vi "Initialization_UI.vi"(8 "error in (no error)":errorcluster, 11 "ZenGage v3.0 UI in":refnum<class "ZenGage v3.0 UI.lvclass">) -> (0 "error out":errorcluster, 3 "ZenGage v3.0 UI out":refnum<class "ZenGage v3.0 UI.lvclass">)   [LabVIEW 2015, in "ZenGage v3.0 UI.lvclass"]
uses:
  ZenGage v3.0 UI.lvclass
  ZenGage v3.0 UI.lvclass/ZenGage v3.0 UI.ctl
  <vilib>/Utility/miscctls.llb/LVRowAndColumnTypeDef.ctl
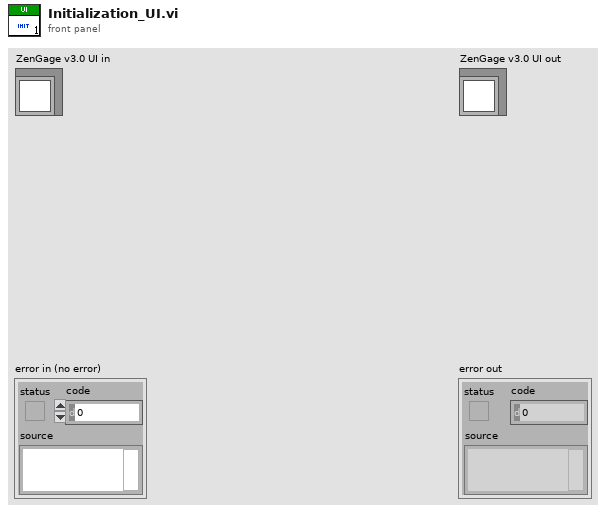
[diagram p1: front panel]
types:
  T1 = enum8{"Enabled", "Disabled", "Disabled and Grayed Out"}
  T2 = enum32{"Edit Tolerance Limits1", "Inspection", "Diagnostics", "Other Diagnostics"}
  T3 = enum32{"Analytics", "Blank", "Diagnostics", "Run", "Edit Tolerance Settings"}
  T4 = typedef "LVRowAndColumnTypeDef.ctl" = cluster{"Row":i32, "Column":i32}
  T5 = typedef "ZenGage v3.0 UI.lvclass/UI JSON read cluster.ctl" = cluster{"UIParameters":cluster{"SpecificationVersion":string, "Title":string, "NumberOfImagesToBeDisplayed":dbl, "ImageCountWindow":dbl, "FontName":string, "FontSize":dbl, "CustomerLogoFilePath":string, "ZentronLogoFilePath":string, "CompatibleSoftwareVersions":string[], "CameraLabelMapping":cluster{"CameraName":string, "ImageLabel":string}[], "ImageIndicatorLayouts":cluster{"NumberOfImageIndicators":dbl, "ImageSpecificData":cluster{"Width":dbl, "Left":dbl, "Top":dbl, "ImagePercentage":cluster{"Height":dbl, "Widthcorrection":i64, "Heightcorrection":i64, "Leftcorrection":dbl, "Topcorrection":dbl}, "StringPercentage":cluster{"Height":dbl, "Widthcorrection":i64, "Heightcorrection":dbl, "Leftcorrection":dbl, "Topcorrection":dbl}}[]}[], "SoftwareButtonLabels":cluster{"SelectLabel":string, "RunLabel":string, "PauseLabel":string, "StopLabel":string}, "DiagnosticsParameters":cluster{"CameraOpticsDiagnostics":cluster{"Label":string, "CameraLabelsList":cluster{"CameraName":string, "ImageLabel":string}[]}, "ArduinoDiagnostics":cluster{"Label":string}, "GuideMotor":cluster{"Label":string}, "ReelerMotor":cluster{"Label":string}, "TowerLamp":cluster{"Label":string}, "TriggerSensor":cluster{"Label":string, "SensorsList":cluster{"SensorName":string, "LabelName":string}[]}, "HardwareButtonDiagnostics":cluster{"Label":string}}, "DieIdParameters":cluster{"DefaultDieId":string, "DieIdsList":string[]}, "EventReasonsList":cluster{"Pause":string[], "Stop":string[], "FailPause":string[], "DefaultEventReason":string}, "StampingMachineIds":string[], "ErrorPopupStrings":cluster{"ErrorCode":string, "ErrorString":string}[]}}
  T6 = cluster{"CameraOpticsDiagnostics":cluster{"Label":string, "CameraLabelsList":cluster{"CameraName":string, "ImageLabel":string}[]}, "ArduinoDiagnostics":cluster{"Label":string}, "GuideMotor":cluster{"Label":string}, "ReelerMotor":cluster{"Label":string}, "TowerLamp":cluster{"Label":string}, "TriggerSensor":cluster{"Label":string, "SensorsList":cluster{"SensorName":string, "LabelName":string}[]}, "HardwareButtonDiagnostics":cluster{"Label":string}}
  T7 = cluster{"Diagnostics names":cluster{"Main diagnostics":string[], "Sub diagnostics names":cluster{"Camera optics":string[], "Trigger sensor":string[]}}, "Diagnostics labels":cluster{"Main diagnostics":string[], "Sub diagnostics names":cluster{"Camera optics":string[], "Trigger sensor":string[]}}}
  T8 = typedef "IMAQ Image.ctl" = refnum<image>
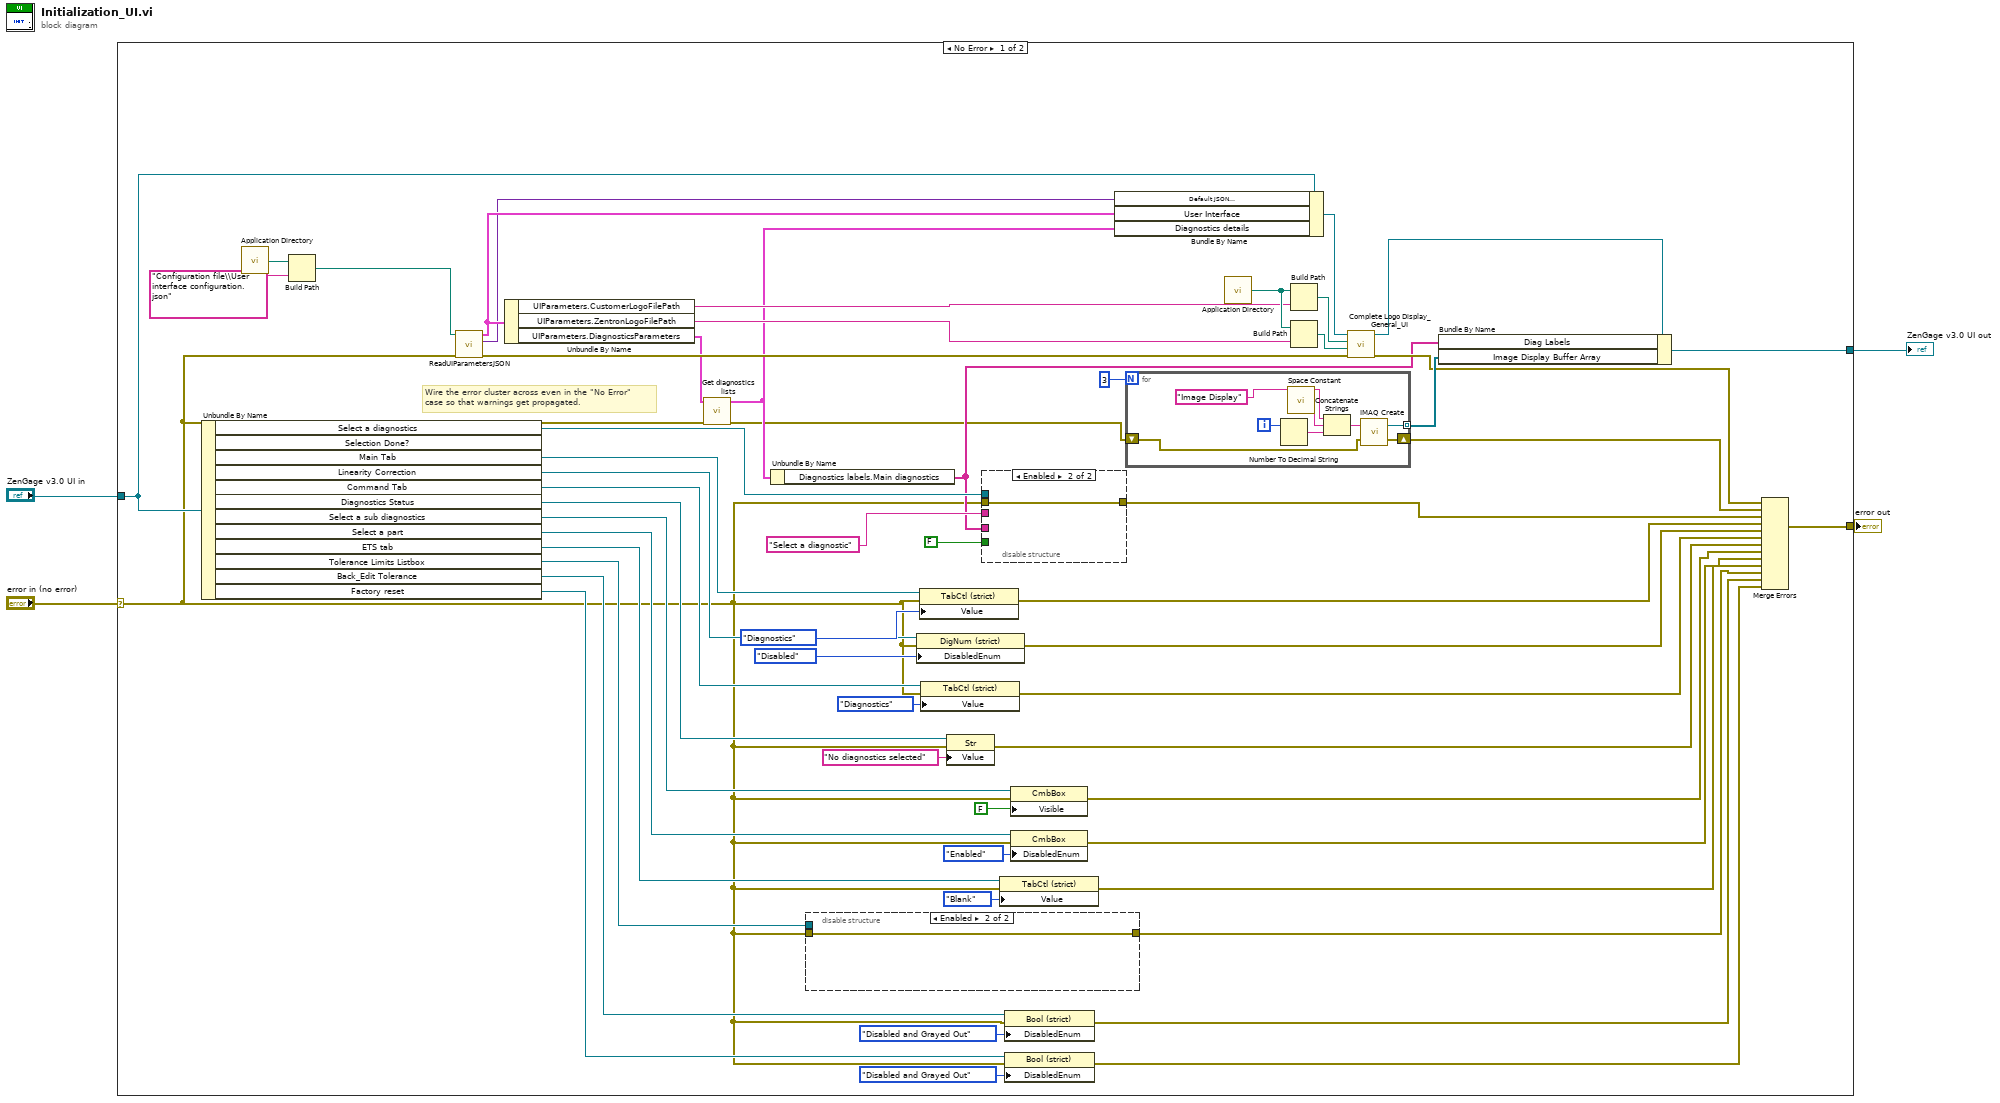
[diagram p0: block diagram]
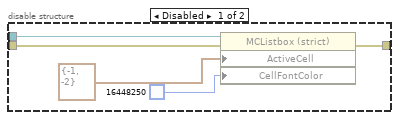
[diagram p2: hidden frame]
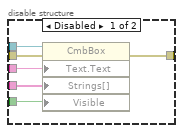
[diagram p3: hidden frame]
diagram:
  n1 = case shown="No Error" "error in (no error)" {
    selector: "error in (no error)" -> [w5 w85]
    tunnel: [w54 w85] -> w3
    tunnel: [w41 w84] -> w1
    tunnel: "ZenGage v3.0 UI in" -> [w51 w84]
    frame No Error {
      # "Wire the error cluster across even in the \"No Error\"\ncase so that warnings get propagated."
      n2 = Unbundle By Name(w51) -> ("Select a diagnostics"=w46:refnum<vi>, "Main Tab"=w48:refnum<vi>, "Linearity Correction"=w44:refnum<vi>, "Command Tab"=w40:refnum<vi>, "Diagnostics Status"=w37:refnum<vi>, "Select a sub diagnostics"=w29:refnum<vi>, "Select a part"=w26:refnum<vi>, "ETS tab"=w17:refnum<vi>, "Tolerance Limits Listbox"=w14:refnum<vi>, "Back_Edit Tolerance"=w13:refnum<vi>, "Factory reset"=w9:refnum<vi>)  [unwired: 1 out]
      n3 = call <vilib>:"Application Directory.vi"() -> ("Application Directory"=w33:path)
      n4 = Build Path(base path=w33, name or relative path="Configuration file\\User interface configuration.json") -> (appended path=w31:path)
      n5 = call "ReadUIParametersJSON.vi"("error in"=w5, "User interface JSON filepath"=w31) -> ("error out"=w56:errorcluster, "JSON Variant out"=w6:variant, "UI JSON"=w30:T5)  [unwired: 7 in]
      n6 = Unbundle By Name(w30) -> ("UIParameters.CustomerLogoFilePath"=w59:string, "UIParameters.ZentronLogoFilePath"=w58:string, "UIParameters.DiagnosticsParameters"=w21:T6)
      n7 = call "Get diagnostics lists.vi"("error in (no error)"=w5, "Diagnostics details"=w21) -> ("error out"=w18:errorcluster, "Diagnostics details"=w19:T7)  [unwired: 8 in]
      n8 = Unbundle By Name(w19) -> ("Diagnostics labels.Main diagnostics"=w20:string[])
      n9 = disable-structure shown="Enabled" {
        disable-tunnel: w14 -> [w67 _]
        disable-tunnel: [w64 w68] -> w11
        disable-tunnel: w5 -> [w63 w68]
        frame Disabled {
          n10 = property class="MCListbox (strict)"(reference=w67, error in=w63, "ActiveCell"=T4 {"Row"=-1, "Column"=-2} ("Active Cell:Active Cell"), "CellFontColor"=u32 16448250) -> (error out=w64:errorcluster)  [unwired: 1 out]
        }
        frame Enabled {
        }
      }
      n11 = property class="DigNum (strict)"(reference=w44, error in=w5, "DisabledEnum"=T1."Disabled" ("Disabled")) -> (error out=w42:errorcluster)  [unwired: 1 out]
      n12 = property class="TabCtl (strict)"(reference=w48, error in=w5, "Value"=T3."Diagnostics") -> (error out=w45:errorcluster)  [unwired: 1 out]
      n13 = property class="TabCtl (strict)"(reference=w40, error in=w5, "Value"=T2."Diagnostics") -> (error out=w38:errorcluster)  [unwired: 1 out]
      n14 = property class="Str"(reference=w37, error in=w5, "Value"="No diagnostics selected") -> (error out=w35:errorcluster)  [unwired: 1 out]
      n15 = disable-structure shown="Enabled" {
        disable-tunnel: "Select a diagnostic" ("Text.Text") -> [w74 _]
        disable-tunnel: [w73 w75] -> w49
        disable-tunnel: w46 -> [w72 _]
        disable-tunnel: FALSE ("Visible") -> [w71 _]
        disable-tunnel: w20 -> [w70 _]
        disable-tunnel: w5 -> [w69 w75]
        frame Disabled {
          n16 = property class="CmbBox"(reference=w72, error in=w69, "Text.Text"=w74, "Strings[]"=w70, "Visible"=w71) -> (error out=w73:errorcluster)  [unwired: 1 out]
        }
        frame Enabled {
        }
      }
      n17 = property class="TabCtl (strict)"(reference=w17, error in=w5, "Value"=enum32{"Display", "Blank"}."Blank") -> (error out=w15:errorcluster)  [unwired: 1 out]
      n18 = property class="Bool (strict)"(reference=w13, error in=w5, "DisabledEnum"=T1."Disabled and Grayed Out" ("Disabled")) -> (error out=w10:errorcluster)  [unwired: 1 out]
      n19 = property class="Bool (strict)"(reference=w9, error in=w5, "DisabledEnum"=T1."Disabled and Grayed Out" ("Disabled")) -> (error out=w7:errorcluster)  [unwired: 1 out]
      n20 = property class="CmbBox"(reference=w29, error in=w5, "Visible"=FALSE) -> (error out=w28:errorcluster)  [unwired: 1 out]
      n21 = property class="CmbBox"(reference=w26, error in=w5, "DisabledEnum"=T1."Enabled" ("Disabled")) -> (error out=w24:errorcluster)  [unwired: 1 out]
      n22 = Bundle By Name(cluster=w51, "Default JSON \nVariant"=w6, "User Interface"=w30, "Diagnostics details"=w19) -> (w57:refnum<class "ZenGage v3.0 UI.lvclass">)
      n23 = for {
        N: 3 -> [_]
        shift-right: [w83] -> w22
        shift-left: w18 -> [w82]
        tunnel: [w76] -> w53 mode=indexing
        i -> [w79]
        n24 = Number To Decimal String(number=w79) -> (decimal integer string=w78:string)  [unwired: 1 in]
        n25 = call <vilib>:"Space Constant.vi"() -> ("String"=w80:string)
        n26 = Concatenate Strings("Image Display" ("Image Name"), w80, w78) -> (w77:string)
        n27 = call "IMAQ Create"("Image Name"=w77, "error in (no error)"=w82) -> ("New Image"=w76:T8, "error out"=w83:errorcluster)  [unwired: 3 in]
      }
      n28 = call <vilib>:"Application Directory.vi"() -> ("Application Directory"=w62:path)
      n29 = Build Path(base path=w62, name or relative path=w59) -> (appended path=w61:path)
      n30 = Build Path(base path=w62, name or relative path=w58) -> (appended path=w60:path)
      n31 = call-dynamic "Complete Logo Display_General_UI.vi"("error in (no error)"=w56, "ZenLogo file path in"=w60, "Customer Company Logo file path in"=w61, "ZenGage v3.0 UI in"=w57) -> ("error out"=w23:errorcluster, "ZenGage v3.0 UI out"=w55:refnum<class "ZenGage v3.0 UI.lvclass">)  [unwired: 6 in]
      n32 = Bundle By Name(cluster=w55, "Diag Labels"=w20, "Image Display Buffer Array"=w53) -> (w41:refnum<class "ZenGage v3.0 UI.lvclass">)
      n33 = Merge Errors(w23, w22, w49, w45, w42, w38, w35, w28, w24, w15, w11, w10, w7) -> (w54:errorcluster)
    }
    frame Error {
    }
  }
  "error out" <- w3
  "ZenGage v3.0 UI out" <- w1
